vi "GL Get Attribute.vi"(8 "error in":errorcluster, 11 "Attribute":u32 format="%.0x") -> (0 "error out":errorcluster, 2 "Value":i32 format="%.0x", 3 "Return":i32)   [LabVIEW 2014, in "LibSDL2.lvlib"]
uses:
  LibSDL2.lvlib
  DLL/SDL2.dll
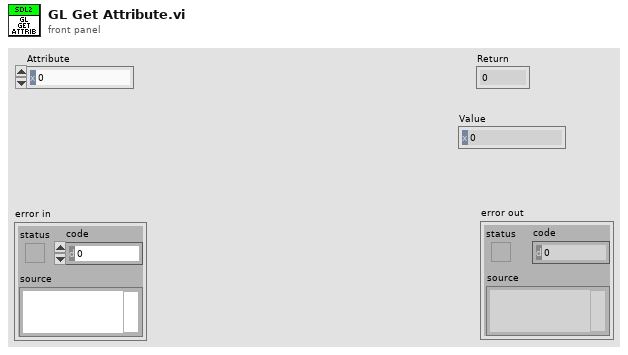
[diagram p1: front panel]
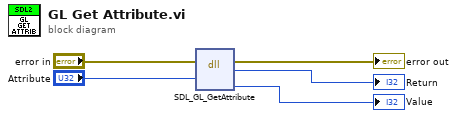
[diagram p0: block diagram]
diagram:
  n1 = dll-call lib="C:/dev/PGS/LabSDL2/Source/LibSDL2 Wrapper/DLL/SDL2.dll" fn="SDL_GL_GetAttribute"(error in="error in", "attribute"="Attribute") -> (error out=→"error out":errorcluster, "return type"=→"Return":i32, "value"=→"Value":i32)  [unwired: 4 in, 1 out]
